vi "DMMportmanager.vi"(0 "port in":variant, 5 "Name":string, 11 "error in (no error)":errorcluster, 12 "Action":enum16{"Read", "Write", "Read All", "Delete"}(ring)) -> (4 "port":variant, 6 "port[]":variant[](array[variant]), 8 "port names[]":string[](array[string]), 15 "error out":errorcluster)   [LabVIEW 2016, in "DMM.lvclass"]
uses:
  DMM.lvclass
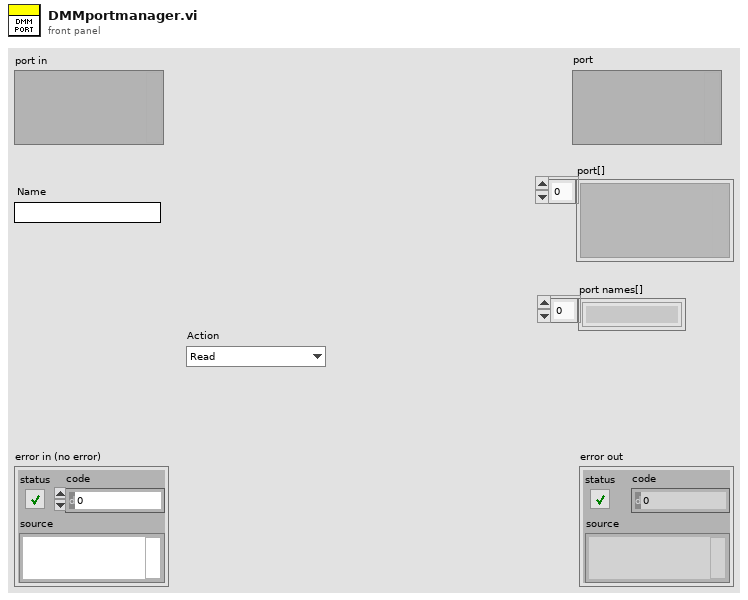
[diagram p1: front panel]
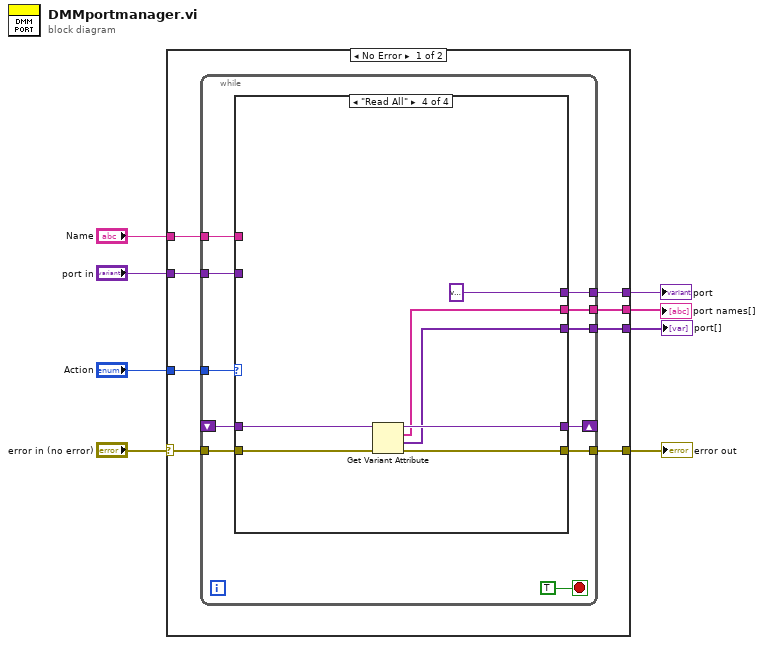
[diagram p0: block diagram]
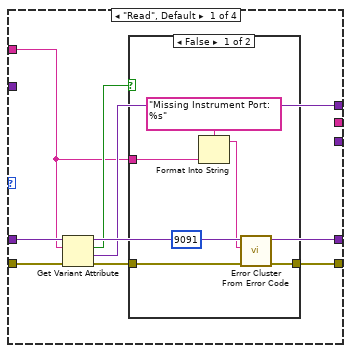
[diagram p2: hidden frame]
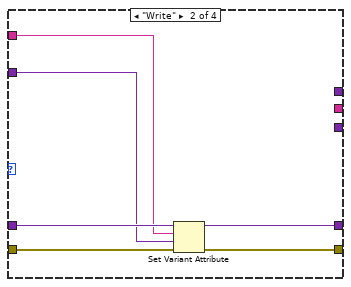
[diagram p4: hidden frame]
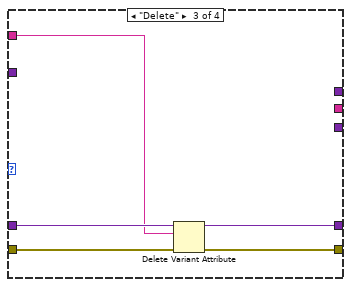
[diagram p5: hidden frame]
diagram:
  n1 = case shown="No Error" "error in (no error)" {
    selector: "error in (no error)" -> [w14 w61]
    tunnel: [w12 w61] -> w7
    tunnel: "port in" -> [w16 _]
    tunnel: "Action" -> [w15 _]
    tunnel: "Name" -> [w13 _]
    tunnel: [w11 _] -> w3
    tunnel: [w10 _] -> w2
    tunnel: [w9 _] -> w1
    frame No Error {
      n2 = while {
        tunnel: w16 -> [w20]
        tunnel: w15 -> [w26]
        tunnel: w14 -> [w25]
        tunnel: w13 -> [w24]
        tunnel: [w23] -> w12
        shift-right: [w22] -> _
        shift-left: _ -> [w21]
        tunnel: [w19] -> w11
        tunnel: [w18] -> w10
        tunnel: [w17] -> w9
        stop <- TRUE stop-if-true
        n3 = case shown="\"Read All\"" w26 {
          tunnel: w25 -> [w34 w48 w53 w60]
          tunnel: w24 -> [w28 w44 w49 _]
          tunnel: [w29 w47 w52 w59] -> w23
          tunnel: [w33 w46 w51 w58] -> w22
          tunnel: w21 -> [w35 w45 w50 w57]
          tunnel: w20 -> [_ w43 _ _]
          tunnel: [w32 _ _ variant] -> w19
          tunnel: [_ _ _ w56] -> w18
          tunnel: [_ _ _ w54] -> w17
          frame "Read", Default {
            n4 = Get Variant Attribute(Variant=w35, name=w28, error in=w34) -> (duplicate Variant=w33:variant, found=w31:bool, value=w32:variant, error out=w30:errorcluster)  [unwired: 1 in]
            n5 = case shown="False" w31 {
              tunnel: w30 -> [w41 w42]
              tunnel: [w40 w42] -> w29
              tunnel: w28 -> [w38 _]
              frame False {
                n6 = Format Into String(format string="Missing Instrument Port: %s" ("error message (\"\")"), w38) -> (resulting string=w36:string)  [unwired: 2 in, 1 out]
                n7 = call <vilib>:"Error Cluster From Error Code.vi"("error in (no error)"=w41, "error message (\"\")"=w36, "error code (0)"=9091) -> ("error out"=w40:errorcluster)  [unwired: 6 in]
              }
              frame True {
              }
            }
          }
          frame "Write" {
            n8 = Set Variant Attribute(Variant=w45, name=w44, value=w43, error in=w48) -> (Variant out=w46:variant, error out=w47:errorcluster)  [unwired: 1 out]
          }
          frame "Delete" {
            n9 = Delete Variant Attribute(4:w53, 6:w49, 7:w50) -> (0:w52:errorcluster, 3:w51:variant)  [unwired: 1 out]
          }
          frame "Read All" {
            n10 = Get Variant Attribute(Variant=w57, error in=w60) -> (duplicate Variant=w58:variant, names=w54:string[], values=w56:variant[], error out=w59:errorcluster)  [unwired: 2 in]
          }
        }
      }
    }
    frame Error {
    }
  }
  "error out" <- w7
  "port" <- w3
  "port[]" <- w2
  "port names[]" <- w1
